vi "Unflatten from string.vi"(2 "Input string":string, 3 "Number of coordinates to extract":i32, 4 "error in (no error)":errorcluster, 5 "queue out":refnum<queue>) -> (0 "Array of coordinates extracted":u8[](array[numeric]), 1 "Array of element extracted\nfrom the array depending on \nthe coordinates given":dbl[](array[numeric]))   [LabVIEW 2021]
panel:
  out "i":i32
  out "index row":u8
  out "index col":u8
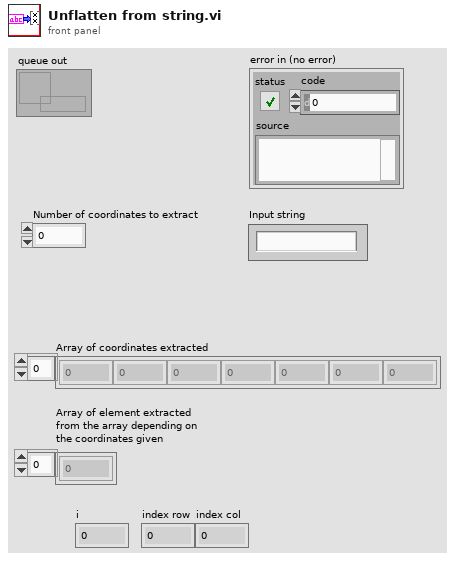
[diagram p1: front panel]
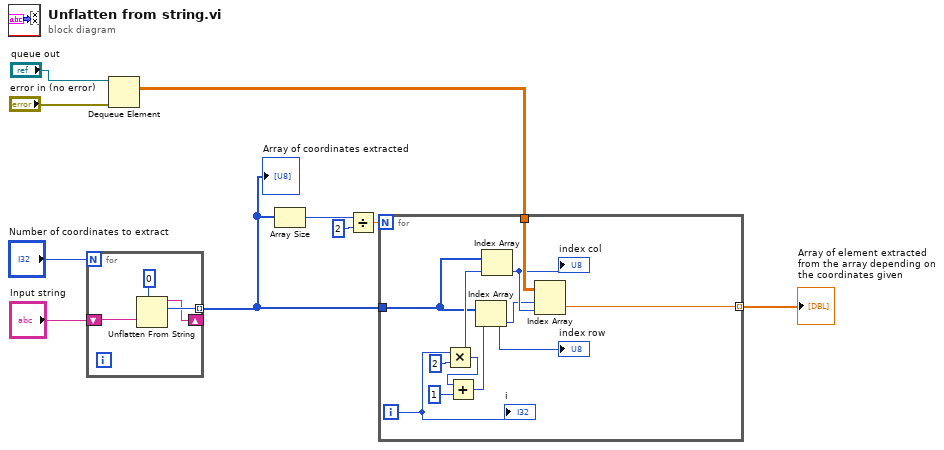
[diagram p0: block diagram]
diagram:
  n1 = for {
    N: "Number of coordinates to extract" -> [_]
    tunnel: [w12] -> w8 mode=indexing
    shift-right: [w11] -> _
    shift-left: "Input string" -> [w13]
    n2 = Unflatten From String(type=u8 0, binary string=w13) -> (rest of the binary string=w11:string, value=w12:u8)  [unwired: 3 in, 1 out]
  }
  "Array of coordinates extracted" <- w8
  n3 = Dequeue Element(queue="queue out", error in (no error)="error in (no error)") -> (element=w2:dbl[][])  [unwired: 1 in, 3 out]
  n4 = Array Size(array=w8) -> (size(s)=w7:i32)
  n5 = Divide(x=w7, y=2) -> (x/y=w5:dbl)
  n6 = for {
    N: w5 -> [_]
    tunnel: w8 -> [w20]
    tunnel: w2 -> [w18]
    tunnel: [w17] -> w1 mode=indexing
    i -> [w19]
    n7 = Multiply(x=w19, y=2) -> (x*y=w21:i32)
    n8 = Add(x=w21, y=1) -> (x+y=w22:i32)
    n9 = Index Array(array=w20, index=w22) -> (element=w15:u8)
    "index row" <- w15
    n10 = Index Array(array=w20, index=w21) -> (element=w16:u8)
    "index col" <- w16
    n11 = Index Array(array=w18, index (row)=w15, index (col)=w16) -> (element=w17:dbl)
    "i" <- w19
  }
  "Array of element extracted\nfrom the array depending on \nthe coordinates given" <- w1
